vi "hellowrold.vi"() -> ()   [LabVIEW 2019]
panel:
  in  "String":string
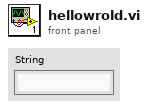
[diagram p1: front panel]
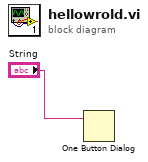
[diagram p0: block diagram]
diagram:
  n1 = One Button Dialog(message="String") -> ()  [unwired: 1 in, 1 out]
